vi "Triangle Top Level VI Solution.vi"() -> ()   [LabVIEW 2015]
uses:
  colors.ctl
  Shape/Shape.lvclass/Shape.ctl
  Shape/Shape.lvclass
panel:
  out "id":string[](array[string])
  out "color":T1[](array[typedef])
  out "perimeter":dbl[](array[numeric])
  out "area":dbl[](array[numeric])
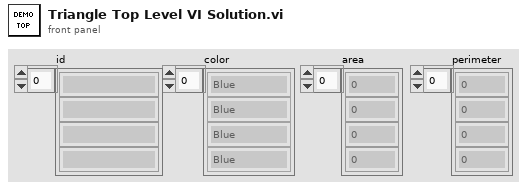
[diagram p1: front panel]
types:
  T1 = typedef "colors.ctl" = enum16{"Blue", "Red", "Green", "Yellow"}
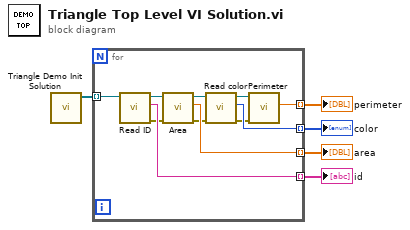
[diagram p0: block diagram]
diagram:
  n1 = call "Triangle Demo Init Solution.vi"() -> ("shape array"=w1:refnum<class "Shape.lvclass">[])  [unwired: 11 in]
  n2 = for {
    tunnel: w1 -> [w16] mode=indexing
    tunnel: [w12] -> w5 mode=indexing
    tunnel: [w11] -> w4 mode=indexing
    tunnel: [w10] -> w3 mode=indexing
    tunnel: [w9] -> w2 mode=indexing
    n3 = call "Read ID.vi"("Shape in"=w16) -> ("error out"=w8:errorcluster, "ID"=w9:string, "Shape out"=w15:refnum<class "Shape.lvclass">)  [unwired: 8 in]
    n4 = call-dynamic "Area.vi"("error in (no error)"=w8, "Shape in"=w15) -> ("error out"=w7:errorcluster, "Numeric"=w12:dbl, "Shape out"=w14:refnum<class "Shape.lvclass">)  [unwired: 7 in]
    n5 = call "Read color.vi"("error in (no error)"=w7, "Shape in"=w14) -> ("error out"=w6:errorcluster, "color"=w10:T1, "Shape out"=w13:refnum<class "Shape.lvclass">)  [unwired: 7 in]
    n6 = call-dynamic "Perimeter.vi"("error in (no error)"=w6, "Shape in"=w13) -> ("perimeter"=w11:dbl)  [unwired: 7 in, 2 out]
  }
  "area" <- w5
  "perimeter" <- w4
  "color" <- w3
  "id" <- w2
